vi "Convert Block Data (SubVI).vi"(10 "Input Array":bool[](array[boolean]), 11 "Bit Depth":u8=8) -> (3 "Output Array":bool[](array[boolean]))   [LabVIEW 2015]
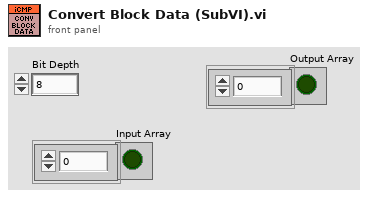
[diagram p1: front panel]
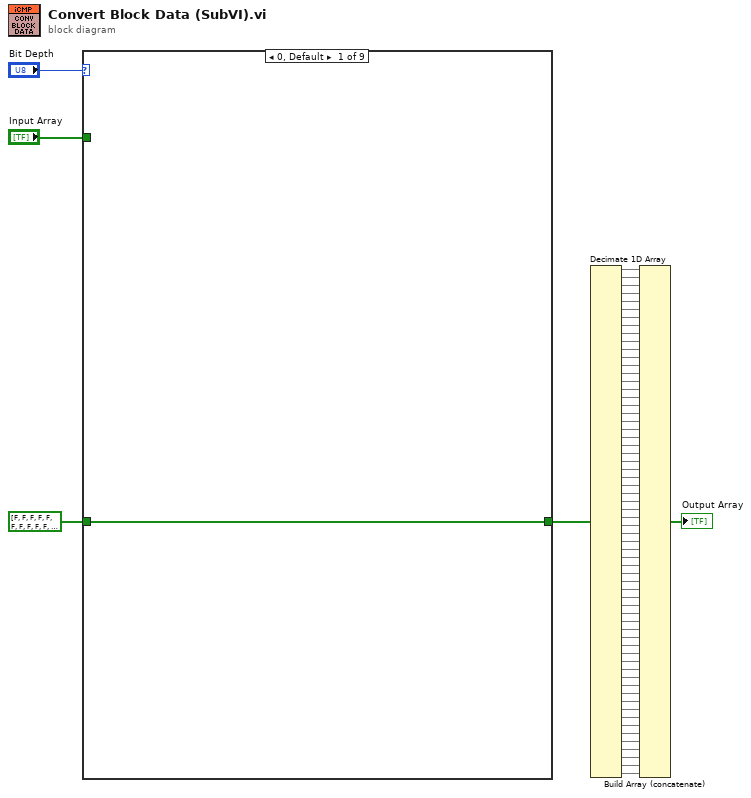
[diagram p0: block diagram]
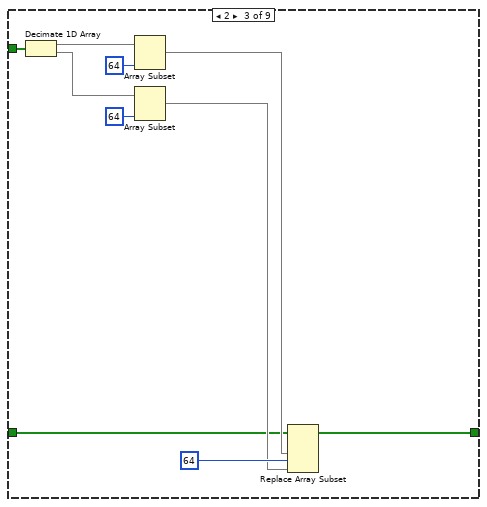
[diagram p3: hidden frame]
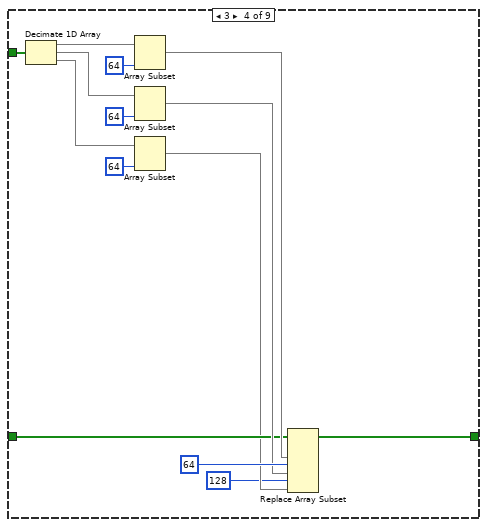
[diagram p4: hidden frame]
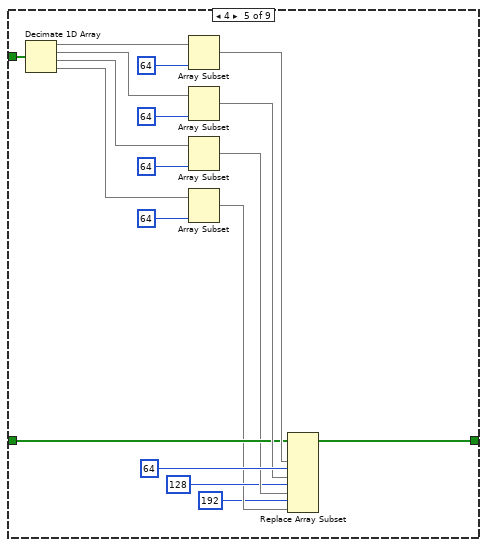
[diagram p5: hidden frame]
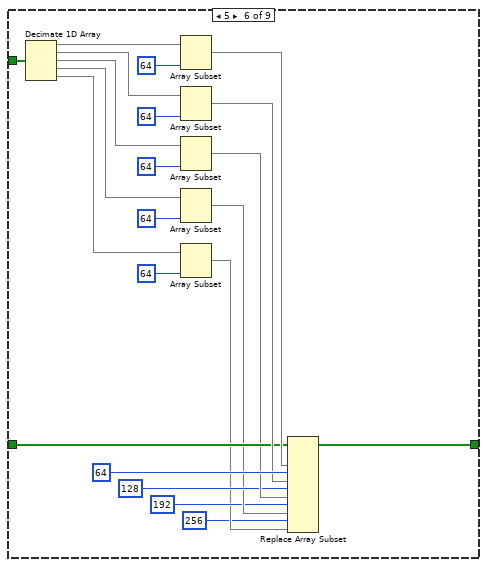
[diagram p6: hidden frame]
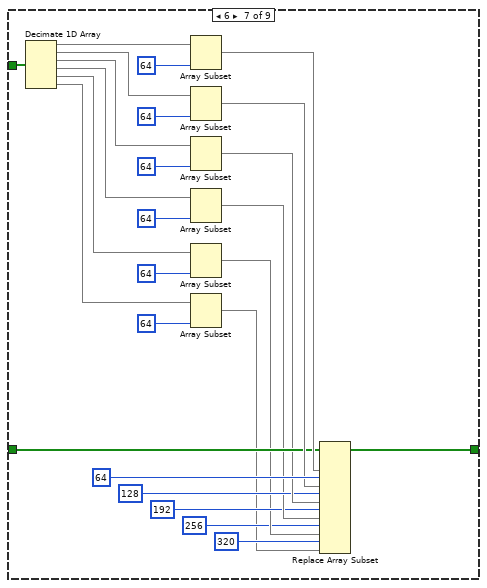
[diagram p7: hidden frame]
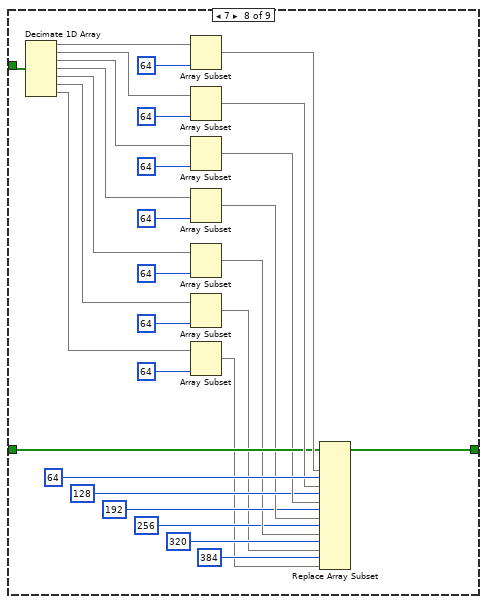
[diagram p8: hidden frame]
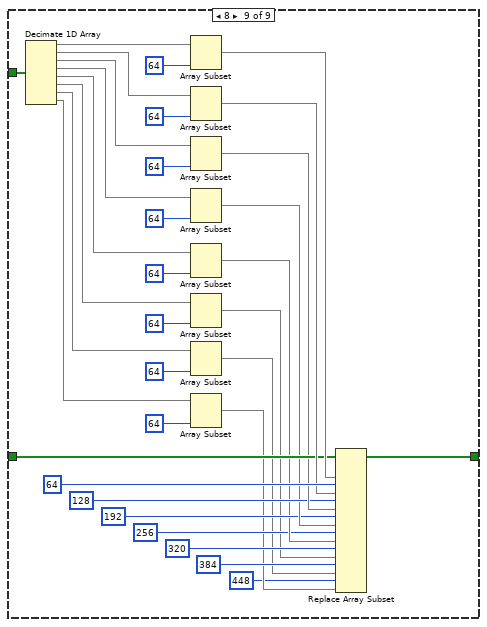
[diagram p9: hidden frame]
diagram:
  n1 = case shown="0, Default" "Bit Depth" {
    tunnel: "Input Array" -> [_ w71 w73 w88 w106 w128 w154 w184 w218]
    tunnel: [w70 w71 w72 w87 w105 w127 w153 w183 w217] -> w68
    tunnel: bool[] [FALSE, FALSE, FALSE, FALSE, FALSE, FALSE, FALSE, FALSE, FALSE, FALSE, FALSE, FALSE, FALSE, FALSE, FALSE, FALSE, FALSE, FALSE, FALSE, FALSE, FALSE, FALSE, FALSE, FALSE, FALSE, FALSE, FALSE, FALSE, FALSE, FALSE, FALSE, FALSE, FALSE, FALSE, FALSE, FALSE, FALSE, FALSE, FALSE, FALSE, FALSE, FALSE, FALSE, FALSE, FALSE, FALSE, FALSE, FALSE, FALSE, FALSE, FALSE, FALSE, FALSE, FALSE, FALSE, FALSE, FALSE, FALSE, FALSE, FALSE, FALSE, FALSE, FALSE, FALSE, FALSE, FALSE, FALSE, FALSE, FALSE, FALSE, FALSE, FALSE, FALSE, FALSE, FALSE, FALSE, FALSE, FALSE, FALSE, FALSE, FALSE, FALSE, FALSE, FALSE, FALSE, FALSE, FALSE, FALSE, FALSE, FALSE, FALSE, FALSE, FALSE, FALSE, FALSE, FALSE, FALSE, FALSE, FALSE, FALSE, FALSE, FALSE, FALSE, FALSE, FALSE, FALSE, FALSE, FALSE, FALSE, FALSE, FALSE, FALSE, FALSE, FALSE, FALSE, FALSE, FALSE, FALSE, FALSE, FALSE, FALSE, FALSE, FALSE, FALSE, FALSE, FALSE, FALSE, FALSE, FALSE, FALSE, FALSE, FALSE, FALSE, FALSE, FALSE, FALSE, FALSE, FALSE, FALSE, FALSE, FALSE, FALSE, FALSE, FALSE, FALSE, FALSE, FALSE, FALSE, FALSE, FALSE, FALSE, FALSE, FALSE, FALSE, FALSE, FALSE, FALSE, FALSE, FALSE, FALSE, FALSE, FALSE, FALSE, FALSE, FALSE, FALSE, FALSE, FALSE, FALSE, FALSE, FALSE, FALSE, FALSE, FALSE, FALSE, FALSE, FALSE, FALSE, FALSE, FALSE, FALSE, FALSE, FALSE, FALSE, FALSE, FALSE, FALSE, FALSE, FALSE, FALSE, FALSE, FALSE, FALSE, FALSE, FALSE, FALSE, FALSE, FALSE, FALSE, FALSE, FALSE, FALSE, FALSE, FALSE, FALSE, FALSE, FALSE, FALSE, FALSE, FALSE, FALSE, FALSE, FALSE, FALSE, FALSE, FALSE, FALSE, FALSE, FALSE, FALSE, FALSE, FALSE, FALSE, FALSE, FALSE, FALSE, FALSE, FALSE, FALSE, FALSE, FALSE, FALSE, FALSE, FALSE, FALSE, FALSE, FALSE, FALSE, FALSE, FALSE, FALSE, FALSE, FALSE, FALSE, FALSE, FALSE, FALSE, FALSE, FALSE, FALSE, FALSE, FALSE, FALSE, FALSE, FALSE, FALSE, FALSE, FALSE, FALSE, FALSE, FALSE, FALSE, FALSE, FALSE, FALSE, FALSE, FALSE, FALSE, FALSE, FALSE, FALSE, FALSE, FALSE, FALSE, FALSE, FALSE, FALSE, FALSE, FALSE, FALSE, FALSE, FALSE, FALSE, FALSE, FALSE, FALSE, FALSE, FALSE, FALSE, FALSE, FALSE, FALSE, FALSE, FALSE, FALSE, FALSE, FALSE, FALSE, FALSE, FALSE, FALSE, FALSE, FALSE, FALSE, FALSE, FALSE, FALSE, FALSE, FALSE, FALSE, FALSE, FALSE, FALSE, FALSE, FALSE, FALSE, FALSE, FALSE, FALSE, FALSE, FALSE, FALSE, FALSE, FALSE, FALSE, FALSE, FALSE, FALSE, FALSE, FALSE, FALSE, FALSE, FALSE, FALSE, FALSE, FALSE, FALSE, FALSE, FALSE, FALSE, FALSE, FALSE, FALSE, FALSE, FALSE, FALSE, FALSE, FALSE, FALSE, FALSE, FALSE, FALSE, FALSE, FALSE, FALSE, FALSE, FALSE, FALSE, FALSE, FALSE, FALSE, FALSE, FALSE, FALSE, FALSE, FALSE, FALSE, FALSE, FALSE, FALSE, FALSE, FALSE, FALSE, FALSE, FALSE, FALSE, FALSE, FALSE, FALSE, FALSE, FALSE, FALSE, FALSE, FALSE, FALSE, FALSE, FALSE, FALSE, FALSE, FALSE, FALSE, FALSE, FALSE, FALSE, FALSE, FALSE, FALSE, FALSE, FALSE, FALSE, FALSE, FALSE, FALSE, FALSE, FALSE, FALSE, FALSE, FALSE, FALSE, FALSE, FALSE, FALSE, FALSE, FALSE, FALSE, FALSE, FALSE, FALSE, FALSE, FALSE, FALSE, FALSE, FALSE, FALSE, FALSE, FALSE, FALSE, FALSE, FALSE, FALSE, FALSE, FALSE, FALSE, FALSE, FALSE, FALSE, FALSE, FALSE, FALSE, FALSE, FALSE, FALSE, FALSE, FALSE, FALSE, FALSE, FALSE, FALSE, FALSE, FALSE, FALSE, FALSE, FALSE, FALSE, FALSE, FALSE, FALSE, FALSE, FALSE, FALSE, FALSE, FALSE, FALSE, FALSE, FALSE, FALSE, FALSE, FALSE, FALSE, FALSE, FALSE, FALSE, FALSE, FALSE, FALSE, FALSE, FALSE, FALSE, FALSE, FALSE, FALSE, FALSE, FALSE, FALSE, FALSE, FALSE, FALSE, FALSE, FALSE, FALSE, FALSE, FALSE, FALSE, FALSE, FALSE, FALSE, FALSE, FALSE, FALSE, FALSE, FALSE, FALSE, FALSE, FALSE, FALSE, FALSE, FALSE, FALSE, FALSE, FALSE, FALSE, FALSE] ("initialized array") -> [w70 _ w74 w89 w107 w129 w155 w185 w219]
    frame 0, Default {
    }
    frame 1 {
    }
    frame 2 {
      n2 = Decimate 1D Array(w73) -> (w81:bool[], w79:bool[])
      n3 = Array Subset(array=w81, length=64 ("index")) -> (w78:bool[])  [unwired: 1 in]
      n4 = Array Subset(array=w79, length=64 ("index")) -> (w77:bool[])  [unwired: 1 in]
      n5 = Replace Array Subset(array=w74, new element #1=w78, new element #2=w77, index #2=64 ("index")) -> (w72:bool[])  [unwired: 1 in]
    }
    frame 3 {
      n6 = Decimate 1D Array(w88) -> (w95:bool[], w85:bool[], w82:bool[])
      n7 = Array Subset(array=w95, length=64 ("index")) -> (w93:bool[])  [unwired: 1 in]
      n8 = Array Subset(array=w85, length=64 ("index")) -> (w92:bool[])  [unwired: 1 in]
      n9 = Array Subset(array=w82, length=64 ("index")) -> (w84:bool[])  [unwired: 1 in]
      n10 = Replace Array Subset(array=w89, new element #1=w93, new element #2=w92, index #2=64 ("index"), new element #3=w84, index #3=128 ("index")) -> (w87:bool[])  [unwired: 1 in]
    }
    frame 4 {
      n11 = Decimate 1D Array(w106) -> (w113:bool[], w103:bool[], w100:bool[], w98:bool[])
      n12 = Array Subset(array=w113, length=64 ("index")) -> (w111:bool[])  [unwired: 1 in]
      n13 = Array Subset(array=w103, length=64 ("index")) -> (w110:bool[])  [unwired: 1 in]
      n14 = Array Subset(array=w100, length=64 ("index")) -> (w102:bool[])  [unwired: 1 in]
      n15 = Array Subset(array=w98, length=64 ("index")) -> (w97:bool[])  [unwired: 1 in]
      n16 = Replace Array Subset(array=w107, new element #1=w111, new element #2=w110, index #2=64 ("index"), new element #3=w102, index #3=128 ("index"), new element #4=w97, index #4=192 ("index")) -> (w105:bool[])  [unwired: 1 in]
    }
    frame 5 {
      n17 = Decimate 1D Array(w128) -> (w135:bool[], w125:bool[], w122:bool[], w120:bool[], w116:bool[])
      n18 = Array Subset(array=w135, length=64 ("index")) -> (w133:bool[])  [unwired: 1 in]
      n19 = Array Subset(array=w125, length=64 ("index")) -> (w132:bool[])  [unwired: 1 in]
      n20 = Array Subset(array=w122, length=64 ("index")) -> (w124:bool[])  [unwired: 1 in]
      n21 = Array Subset(array=w120, length=64 ("index")) -> (w119:bool[])  [unwired: 1 in]
      n22 = Array Subset(array=w116, length=64 ("index")) -> (w115:bool[])  [unwired: 1 in]
      n23 = Replace Array Subset(array=w129, new element #1=w133, new element #2=w132, index #2=64 ("index"), new element #3=w124, index #3=128 ("index"), new element #4=w119, index #4=192 ("index"), new element #5=w115, index #5=256 ("index")) -> (w127:bool[])  [unwired: 1 in]
    }
    frame 6 {
      n24 = Decimate 1D Array(w154) -> (w161:bool[], w151:bool[], w148:bool[], w146:bool[], w138:bool[], w137:bool[])
      n25 = Array Subset(array=w161, length=64 ("index")) -> (w159:bool[])  [unwired: 1 in]
      n26 = Array Subset(array=w151, length=64 ("index")) -> (w158:bool[])  [unwired: 1 in]
      n27 = Array Subset(array=w148, length=64 ("index")) -> (w150:bool[])  [unwired: 1 in]
      n28 = Array Subset(array=w146, length=64 ("index")) -> (w145:bool[])  [unwired: 1 in]
      n29 = Array Subset(array=w138, length=64 ("index")) -> (w142:bool[])  [unwired: 1 in]
      n30 = Array Subset(array=w137, length=64 ("index")) -> (w136:bool[])  [unwired: 1 in]
      n31 = Replace Array Subset(array=w155, new element #1=w159, new element #2=w158, index #2=64 ("index"), new element #3=w150, index #3=128 ("index"), new element #4=w145, index #4=192 ("index"), new element #5=w142, index #5=256 ("index"), new element #6=w136, index #6=320 ("index")) -> (w153:bool[])  [unwired: 1 in]
    }
    frame 7 {
      n32 = Decimate 1D Array(w184) -> (w191:bool[], w181:bool[], w178:bool[], w176:bool[], w168:bool[], w167:bool[], w163:bool[])
      n33 = Array Subset(array=w191, length=64 ("index")) -> (w189:bool[])  [unwired: 1 in]
      n34 = Array Subset(array=w181, length=64 ("index")) -> (w188:bool[])  [unwired: 1 in]
      n35 = Array Subset(array=w178, length=64 ("index")) -> (w180:bool[])  [unwired: 1 in]
      n36 = Array Subset(array=w176, length=64 ("index")) -> (w175:bool[])  [unwired: 1 in]
      n37 = Array Subset(array=w168, length=64 ("index")) -> (w172:bool[])  [unwired: 1 in]
      n38 = Array Subset(array=w167, length=64 ("index")) -> (w166:bool[])  [unwired: 1 in]
      n39 = Array Subset(array=w163, length=64 ("index")) -> (w162:bool[])  [unwired: 1 in]
      n40 = Replace Array Subset(array=w185, new element #1=w189, new element #2=w188, index #2=64 ("index"), new element #3=w180, index #3=128 ("index"), new element #4=w175, index #4=192 ("index"), new element #5=w172, index #5=256 ("index"), new element #6=w166, index #6=320 ("index"), new element #7=w162, index #7=384 ("index")) -> (w183:bool[])  [unwired: 1 in]
    }
    frame 8 {
      n41 = Decimate 1D Array(w218) -> (w225:bool[], w215:bool[], w212:bool[], w210:bool[], w202:bool[], w201:bool[], w197:bool[], w194:bool[])
      n42 = Array Subset(array=w225, length=64 ("index")) -> (w223:bool[])  [unwired: 1 in]
      n43 = Array Subset(array=w215, length=64 ("index")) -> (w222:bool[])  [unwired: 1 in]
      n44 = Array Subset(array=w212, length=64 ("index")) -> (w214:bool[])  [unwired: 1 in]
      n45 = Array Subset(array=w210, length=64 ("index")) -> (w209:bool[])  [unwired: 1 in]
      n46 = Array Subset(array=w202, length=64 ("index")) -> (w206:bool[])  [unwired: 1 in]
      n47 = Array Subset(array=w201, length=64 ("index")) -> (w200:bool[])  [unwired: 1 in]
      n48 = Array Subset(array=w197, length=64 ("index")) -> (w196:bool[])  [unwired: 1 in]
      n49 = Array Subset(array=w194, length=64 ("index")) -> (w193:bool[])  [unwired: 1 in]
      n50 = Replace Array Subset(array=w219, new element #1=w223, new element #2=w222, index #2=64 ("index"), new element #3=w214, index #3=128 ("index"), new element #4=w209, index #4=192 ("index"), new element #5=w206, index #5=256 ("index"), new element #6=w200, index #6=320 ("index"), new element #7=w196, index #7=384 ("index"), new element #8=w193, index #8=448 ("index")) -> (w217:bool[])  [unwired: 1 in]
    }
  }
  n51 = Decimate 1D Array(w68) -> (w67:bool[], w66:bool[], w65:bool[], w64:bool[], w63:bool[], w62:bool[], w61:bool[], w60:bool[], w59:bool[], w58:bool[], w57:bool[], w56:bool[], w55:bool[], w54:bool[], w53:bool[], w52:bool[], w51:bool[], w50:bool[], w49:bool[], w48:bool[], w47:bool[], w46:bool[], w45:bool[], w44:bool[], w43:bool[], w42:bool[], w41:bool[], w40:bool[], w39:bool[], w38:bool[], w37:bool[], w36:bool[], w35:bool[], w34:bool[], w33:bool[], w32:bool[], w31:bool[], w30:bool[], w29:bool[], w28:bool[], w27:bool[], w26:bool[], w25:bool[], w24:bool[], w23:bool[], w22:bool[], w21:bool[], w20:bool[], w19:bool[], w18:bool[], w17:bool[], w16:bool[], w15:bool[], w14:bool[], w13:bool[], w12:bool[], w11:bool[], w10:bool[], w9:bool[], w8:bool[], w7:bool[], w6:bool[], w5:bool[], w4:bool[])
  n52 = Build Array (concatenate)(w67, w66, w65, w64, w63, w62, w61, w60, w59, w58, w57, w56, w55, w54, w53, w52, w51, w50, w49, w48, w47, w46, w45, w44, w43, w42, w41, w40, w39, w38, w37, w36, w35, w34, w33, w32, w31, w30, w29, w28, w27, w26, w25, w24, w23, w22, w21, w20, w19, w18, w17, w16, w15, w14, w13, w12, w11, w10, w9, w8, w7, w6, w5, w4) -> (→"Output Array":bool[])
